vi "Itest.vi"() -> ()   [LabVIEW 2024]
uses:
  <vilib>/Analysis/baseanly.llb/Mean (DBL).vi
  <instrlib>/EFmeter/EFmeter.lvlib
  <vilib>/Analysis/NI_AALBase.lvlib
  BK Precision 8500B Series/BK Precision 8500B Series.lvlib
  Keithley DMM6500 DAQ6500 Series.lvlib
panel:
  in  "VISA DMM":refnum<visa-resource-name>
  in  "Zdroj":u16(ring) items=["Manualni", "K 2200"]
  out "error out 2":errorcluster
  in  "VISA EFmeter":refnum<visa-resource-name>
  out "R_out":dbl
  in  "file path (use dialog)":path
  in  "Prodleva mezi vzorky":u32
  out "napeti":dbl=2.5
  in  "velikost kroku":dbl
  in  "start":dbl
  in  "Prumerovani":bool
  in  "Vzorku na krokù":u16 max=100 step=1
  out "XY Graph 2":cluster{"X":dbl[], "Y":dbl[]}[](graph)
  in  "Pocet kroku":i32
  in  "Clear":bool
  in  "Uložit data":bool
  in  "Start":bool
  in  "VISA ZATEZ":refnum<visa-resource-name>
  in  "stop":bool
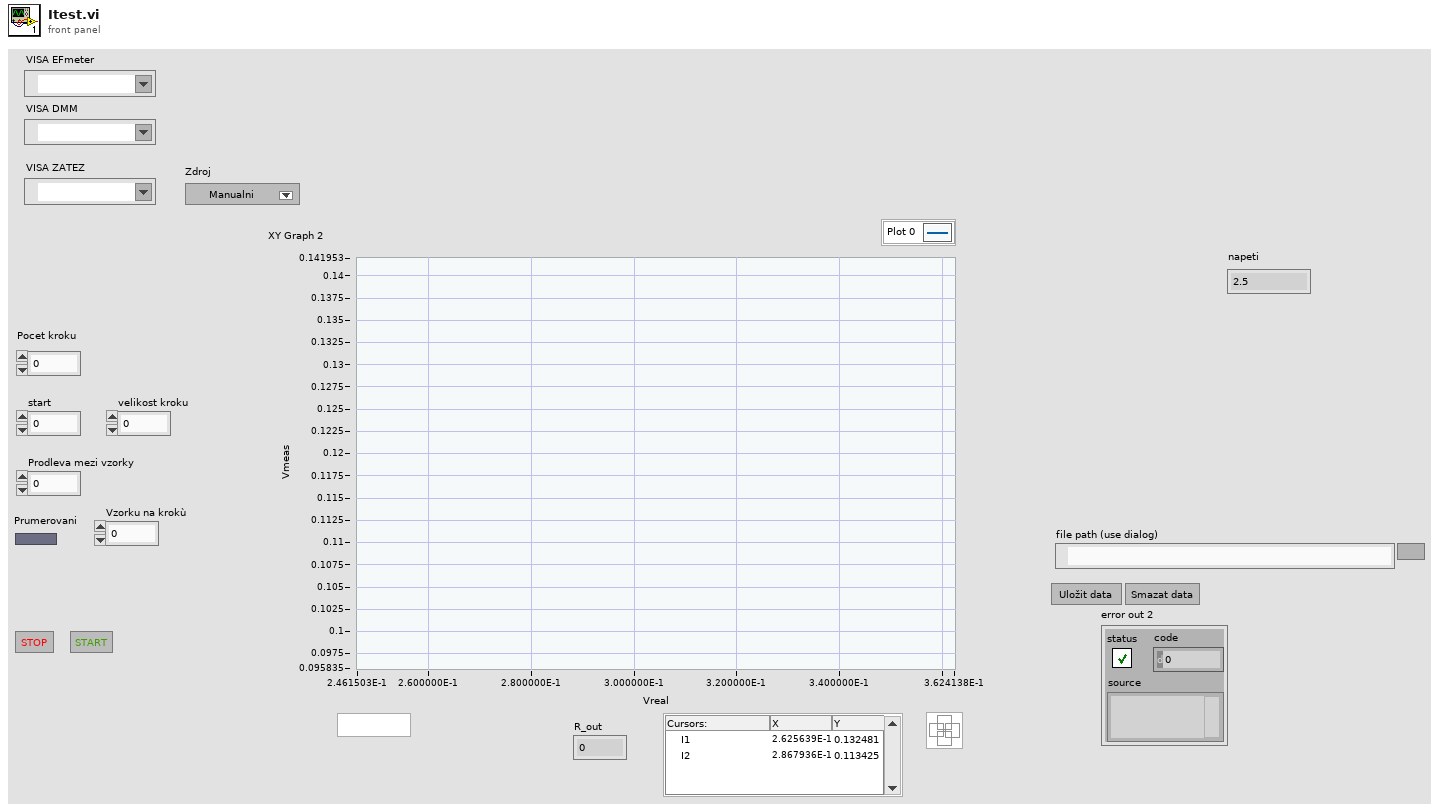
[diagram p1: front panel]
types:
  T1 = enum16{"init", "wait", "graph", "meas", "change_load", "init_measurment", "save", "clear"}
  T2 = typedef "LVCursorListTypeDef.ctl" = cluster{"Name":string, "Color":u32, "Style":u8, "Point Style":u8, "Name Visible":bool, "Allow Drag":bool, "Cursor Mode":u32, "Plot":i32, "Index":i32, "Position":cluster{"X":dbl, "Y":dbl}, "X Scale":u32, "Y Scale":u32, "Watch Plots":i32[], "Watch All Plots":bool, "Plot Area":i32, "Label Offset":cluster{"X":dbl, "Y":dbl}}[]
  T3 = cluster{"Name":string, "Color":u32, "Style":u8, "Point Style":u8, "Name Visible":bool, "Allow Drag":bool, "Cursor Mode":u32, "Plot":i32, "Index":i32, "Position":cluster{"X":dbl, "Y":dbl}, "X Scale":u32, "Y Scale":u32, "Watch Plots":i32[], "Watch All Plots":bool, "Plot Area":i32, "Label Offset":cluster{"X":dbl, "Y":dbl}}
  T4 = enum16{"open", "replace", "create", "open or create", "replace or create", "replace or create with confirmation"}
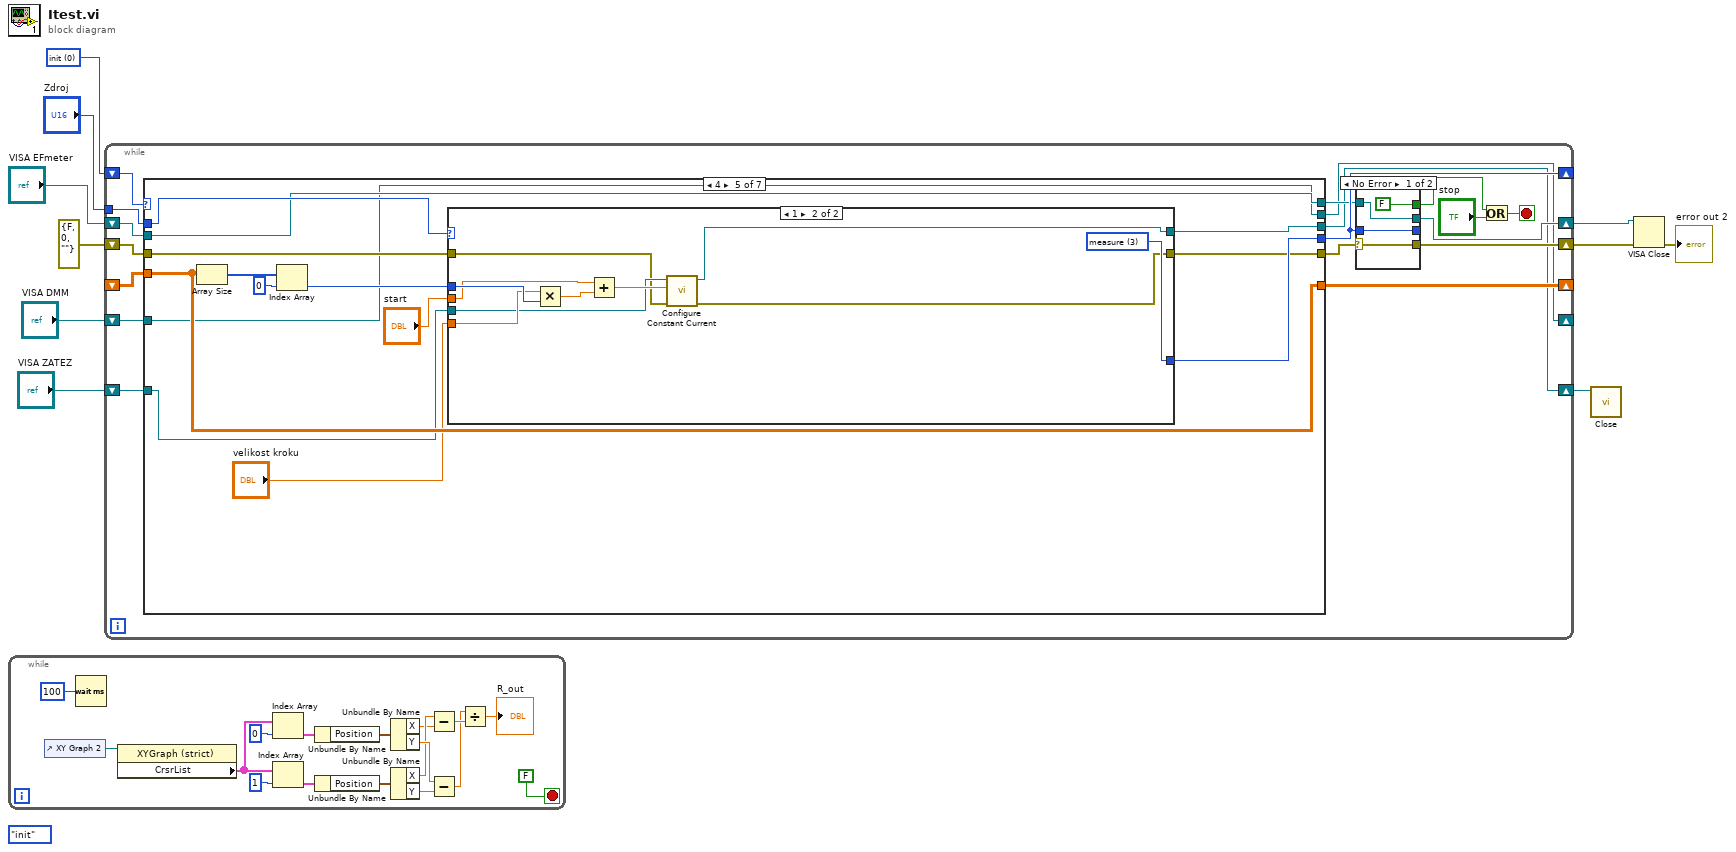
[diagram p0: block diagram]
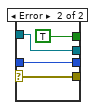
[diagram p2: hidden frame]
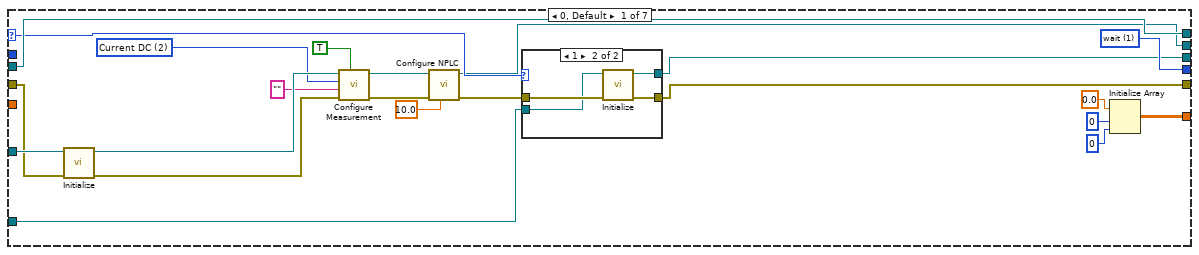
[diagram p3: hidden frame]
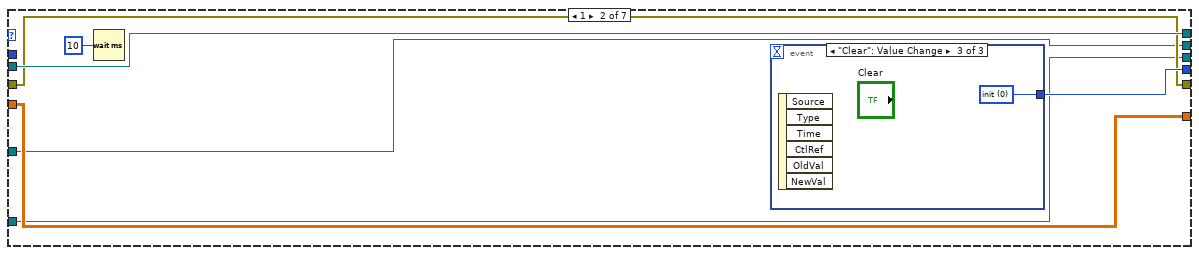
[diagram p5: hidden frame]
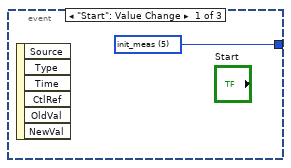
[diagram p6: hidden frame]
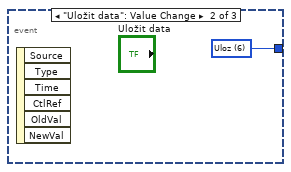
[diagram p7: hidden frame]
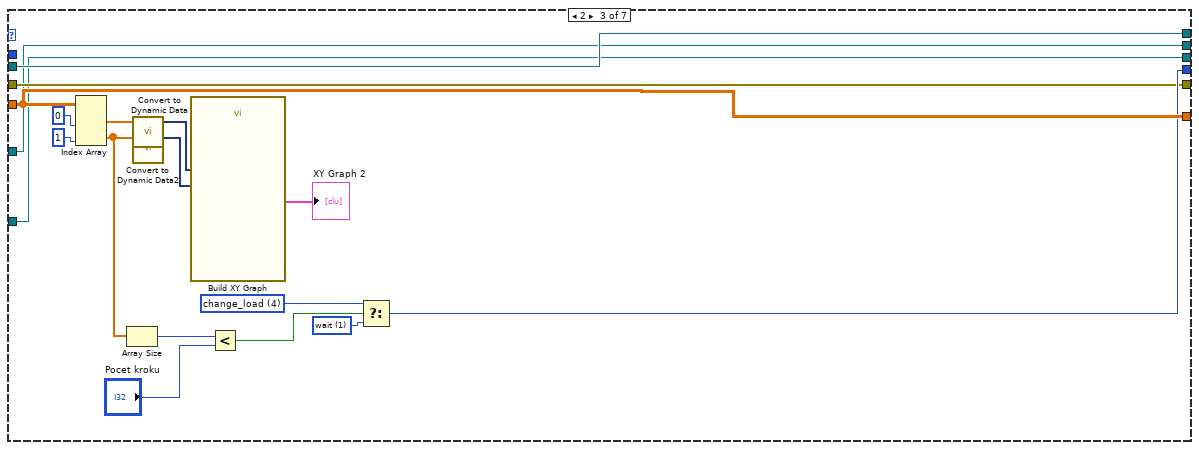
[diagram p8: hidden frame]
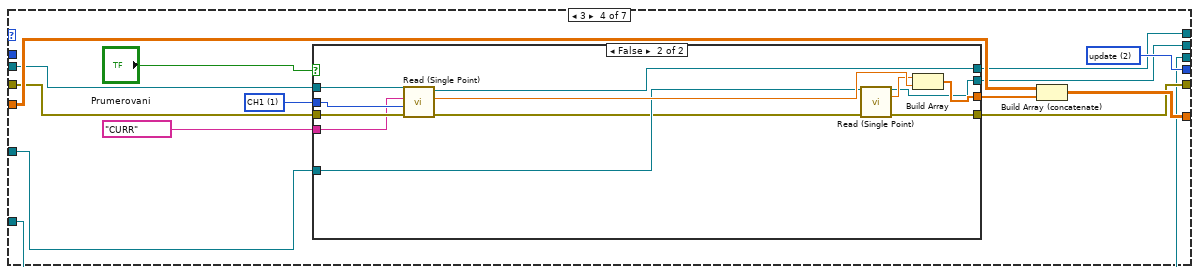
[diagram p9: hidden frame]
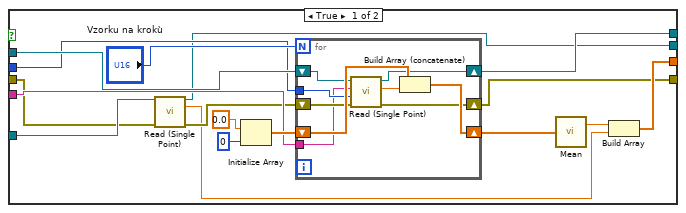
[diagram p10: hidden frame]
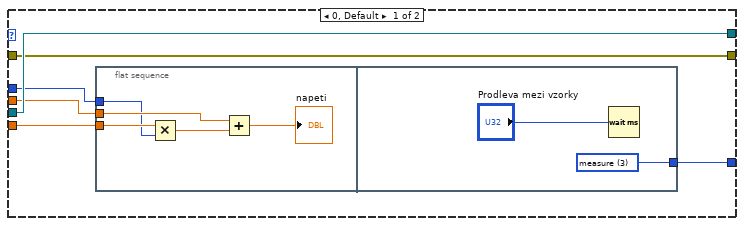
[diagram p11: hidden frame]
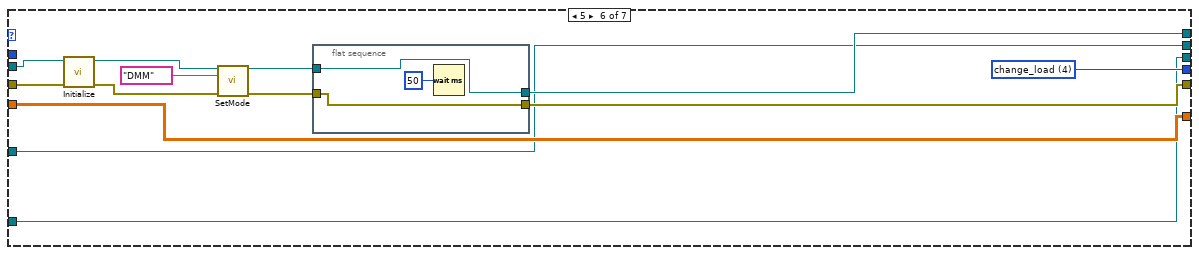
[diagram p12: hidden frame]
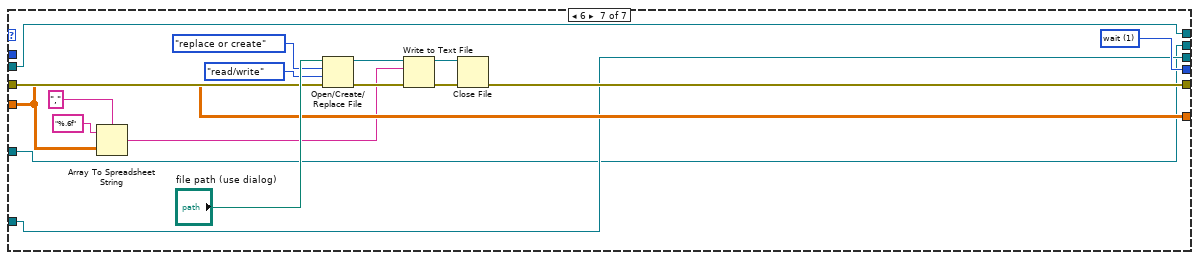
[diagram p13: hidden frame]
diagram:
  (unwired) T1."init"
  w10 = u16 0 items=["init", "wait", "update", "measure", "change_load", "init_meas", "Uloz", "clear"]
  n1 = while {
    stop <- FALSE stop-if-true
    n2 = control-ref of="XY Graph 2"() -> (w25:refnum<vi>)
    n3 = Wait (ms)(milliseconds to wait=u32 100) -> ()  [unwired: 1 out]
    n4 = property class="XYGraph (strict)"(reference=w25) -> ("CrsrList"=w20:T2)  [unwired: 1 in, 2 out]
    n5 = Index Array(array=w20, index=0) -> (element=w26:T3)
    n6 = Index Array(array=w20, index=1) -> (element=w22:T3)
    n7 = Unbundle By Name(w26) -> ("Position"=w27:cluster{"X":dbl, "Y":dbl})
    n8 = Unbundle By Name(w22) -> ("Position"=w23:cluster{"X":dbl, "Y":dbl})
    n9 = Unbundle By Name(w27) -> ("X"=w11:dbl, "Y"=w18:dbl)
    n10 = Unbundle By Name(w23) -> ("X"=w12:dbl, "Y"=w19:dbl)
    n11 = Subtract(x=w12, y=w11) -> (x-y=w14:dbl)
    n12 = Subtract(x=w18, y=w19) -> (x-y=w13:dbl)
    n13 = Divide(x=w13, y=w14) -> (x/y=→"R_out":dbl)
  }
  n14 = while {
    shift-right: [w45] -> _
    shift-left: _ -> [w44]
    shift-right: [w40] -> _
    shift-left: w10 -> [w43]
    shift-right: [w37] -> w6
    shift-left: "VISA EFmeter" -> [w42]
    shift-right: [w36] -> w5
    shift-left: errorcluster {"status"=FALSE, "code"=0, "source"=""} ("error in (no error)") -> [w41]
    tunnel: "Zdroj" -> [w32]
    shift-right: [w31] -> w3
    shift-left: "VISA ZATEZ" -> [w30]
    shift-right: [w28] -> _
    shift-left: "VISA DMM" -> [w29]
    stop <- w34 stop-if-true
    n15 = case shown="4" w43 {
      selector: w43 -> [w69 _ _ _ _ _ _]
      tunnel: [w73 w87 w101 w122 w175 w211 w226] -> w45
      tunnel: w44 -> [_ w87 w101 w123 w175 w211 w226]
      tunnel: [w72 w88 w100 w120 w173 w205 w224] -> w40
      tunnel: [w68 w85 w94 w114 w163 w202 w220] -> w39
      tunnel: [w70 w86 w95 w115 w172 w204 w231] -> w38
      tunnel: w42 -> [w70 w86 w95 w119 w172 w207 w231]
      tunnel: w41 -> [w64 w85 w94 w118 w164 w206 w227]
      tunnel: w32 -> [_ _ _ _ w174 _ _]
      tunnel: [w67 w83 w93 w112 w170 w200 w216] -> w31
      tunnel: w30 -> [w66 w83 w93 w112 w171 w200 w216]
      tunnel: w29 -> [w65 w82 w92 w111 w162 w199 w215]
      tunnel: [w55 w82 w92 w110 w162 w199 w215] -> w28
      frame 0, Default {
        w61 = 2 items=["Voltage DC", "Voltage AC", "Current DC", "Current AC", "Resistance", "4-wire Resistance", "Diode", "Capacitance", "Temperature", "Continuity", "Frequency", "Period", "Voltage Ratio", "Digitize Voltage", "Digitize Current"] ("Function (0: Voltage DC)")
        w72 = u16 1 items=["init", "wait", "update", "measure"]
        n16 = call "Initialize.vi"("error in (no error)"=w64, "VISA resource name"=w65) -> ("error out"=w63:errorcluster, "VISA resource name out"=w62:refnum<visa-resource-name>)  [unwired: 8 in]
        n17 = call "Configure Measurement.vi"("Auto Range (T: Enable)"=TRUE, "error in (no error)"=w63, "Channel List(\"\")"="" ("Channel List(\"\")"), "Function (0: Voltage DC)"=w61, "VISA resource name"=w62) -> ("error out"=w56:errorcluster, "VISA resource name out"=w57:refnum<visa-resource-name>)  [unwired: 5 in]
        n18 = call "Configure NPLC.vi"("Power Line Cycle (1)"=10.0, "error in (no error)"=w56, "VISA resource name"=w57) -> ("error out"=w54:errorcluster, "VISA resource name out"=w55:refnum<visa-resource-name>)  [unwired: 7 in]
        n19 = case shown="1" w69 {
          tunnel: w54 -> [w77 w81]
          tunnel: [w77 w78] -> w68
          tunnel: [w76 w79] -> w67
          tunnel: w66 -> [w76 w80]
          frame 0, Default {
          }
          frame 1 {
            n20 = call "Initialize.vi"("error in (no error)"=w81, "VISA resource name"=w80) -> ("error out"=w78:errorcluster, "VISA resource name out"=w79:refnum<visa-resource-name>)  [unwired: 8 in]
          }
        }
        n21 = Initialize Array(0.0 ("element"), 0 ("dimension size"), 0 ("dimension size")) -> (w73:dbl[][])
      }
      frame 1 {
        n22 = Wait (ms)(milliseconds to wait=u32 10) -> ()  [unwired: 1 out]
        n23 = event shown="[2] \"Clear\": Value Change" {
          selector: _ -> [_ _ _]
          dyn-events: _ -> [_ _ _]
          timeout: _ -> [_ _ _]
          tunnel: [w89 w90 w91] -> w88
          event "Start": Value Change {
            w89 = u16 5 items=["init", "wait", "update", "measure", "change_load", "init_meas"]
            n24 = event-data() -> ()  [unwired: 1 in, 6 out]
          }
          event "Uložit data": Value Change {
            w90 = u16 6 items=["init", "wait", "update", "measure", "change_load", "init_meas", "Uloz"]
            n25 = event-data() -> ()  [unwired: 1 in, 6 out]
          }
          event "Clear": Value Change {
            w91 = u16 0 items=["init", "wait", "update", "measure", "change_load", "init_meas", "Uloz", "clear"]
            n26 = event-data() -> ()  [unwired: 1 in, 6 out]
          }
        }
      }
      frame 2 {
        w96 = u16 4 items=["init", "wait", "update", "measure", "change_load", "init_meas"]
        w102 = u16 1 items=["init", "wait", "update", "measure"]
        n27 = Index Array(array=w101, index (col) #1=0 ("index (row)"), index (col) #2=1 ("index (row)")) -> (element #1=w109:dbl[], element #2=w104:dbl[])  [unwired: 2 in]
        n28 = Array Size(array=w104) -> (size(s)=w106:i32)
        n29 = call "Convert to Dynamic Data"("Array"=w109) -> ("Dynamic Data Type"=w108:dynamicdata)  [unwired: 3 in]
        n30 = call "Convert to Dynamic Data2"("Array"=w104) -> ("Dynamic Data Type"=w107:dynamicdata)  [unwired: 3 in]
        n31 = call "Build XY Graph"("Y Input"=w107, "X Input"=w108) -> ("XY Graph"=→"XY Graph 2":cluster{"X":dbl[], "Y":dbl[]}[])  [unwired: 8 in, 1 out]
        n32 = Less?(x=w106, y="Pocet kroku") -> (x < y?=w105:bool)
        n33 = Select(t=w96, s=w105, f=w102) -> (s? t:f=w100:u16)
      }
      frame 3 {
        w117 = u16 1 items=["CH2"=2, "CH1"=1] ("Ring")
        w120 = u16 2 items=["init", "wait", "update", "measure"]
        n34 = case shown="False" "Prumerovani" {
          tunnel: [w132 w161] -> w121
          tunnel: w119 -> [w136 w160]
          tunnel: w118 -> [w127 w159]
          tunnel: w117 -> [w135 w158]
          tunnel: "CURR" ("Combo Box") -> [w134 w157]
          tunnel: [w131 w152] -> w115
          tunnel: [w130 w153] -> w114
          tunnel: w111 -> [w129 w155]
          tunnel: [w128 w150] -> w110
          frame True {
            n35 = call "Read (Single Point).vi"("VISA resource name"=w129, "error in (no error)"=w127) -> ("VISA resource name out"=w128:refnum<visa-resource-name>, "Measurement"=w125:dbl, "error out"=w126:errorcluster)  [unwired: 11 in]
            n36 = Initialize Array(0.0 ("element"), 0 ("dimension size")) -> (w137:dbl[])
            n37 = for {
              N: "Vzorku na krokù" -> [_]
              shift-right: [w142] -> w131
              shift-left: w136 -> [w148]
              shift-right: [w143] -> w130
              shift-left: w126 -> [w147]
              tunnel: w135 -> [w146]
              tunnel: w134 -> [w145]
              shift-right: [w144] -> w124
              shift-left: w137 -> [w149]
              n38 = call "Read (Single Point).vi"("error in (no error)"=w147, "Ring"=w146, "Combo Box"=w145, "VISA resource name"=w148) -> ("error out"=w143:errorcluster, "Measurement"=w141:dbl, "VISA resource name out"=w142:refnum<visa-resource-name>)  [unwired: 5 in]
              n39 = Build Array (concatenate)(w149, w141) -> (w144:dbl[])
            }
            n40 = call-poly <vilib>:"Mean.vi"("X"=w124) -> ("mean"=w133:dbl)  [unwired: 1 out]
            n41 = Build Array(w133, w125) -> (w132:dbl[])
          }
          frame False {
            n42 = call "Read (Single Point).vi"("error in (no error)"=w159, "Ring"=w158, "Combo Box"=w157, "VISA resource name"=w160) -> ("error out"=w154:errorcluster, "Measurement"=w156:dbl, "VISA resource name out"=w152:refnum<visa-resource-name>)  [unwired: 5 in]
            n43 = call "Read (Single Point).vi"("VISA resource name"=w155, "error in (no error)"=w154) -> ("VISA resource name out"=w150:refnum<visa-resource-name>, "Measurement"=w151:dbl, "error out"=w153:errorcluster)  [unwired: 11 in]
            n44 = Build Array(w151, w156) -> (w161:dbl[])
          }
        }
        n45 = Build Array (concatenate)(w123, w121) -> (w122:dbl[][])
      }
      frame 4 {
        n46 = Array Size(array=w175) -> (size(s)=w165:i32[])
        n47 = Index Array(array=w165, index=0) -> (element=w167:i32)
        n48 = case shown="1" w174 {
          tunnel: [w181 w198] -> w173
          tunnel: w171 -> [w180 w190]
          tunnel: [w180 w193] -> w170
          tunnel: "velikost kroku" -> [w179 w196]
          tunnel: "start" -> [w178 w194]
          tunnel: w167 -> [w177 w197]
          tunnel: w164 -> [w176 w189]
          tunnel: [w176 w192] -> w163
          frame 0, Default {
            n49 = flat-sequence {
              tunnel: w179 -> [w184]
              tunnel: w178 -> [w183]
              tunnel: w177 -> [w182]
              tunnel: [w187] -> w181
              frame #0 {
                n50 = Multiply(x=w184, y=w182) -> (x*y=w186:dbl)
                n51 = Add(x=w183, y=w186) -> (x+y=→"napeti":dbl)
              }
              frame #1 {
                w187 = u16 3 items=["init", "wait", "update", "measure", "change_load", "init_meas"]
                n52 = Wait (ms)(milliseconds to wait="Prodleva mezi vzorky") -> ()  [unwired: 1 out]
              }
            }
          }
          frame 1 {
            w198 = u16 3 items=["init", "wait", "update", "measure", "change_load", "init_meas"]
            n53 = Multiply(x=w196, y=w197) -> (x*y=w195:dbl)
            n54 = Add(x=w194, y=w195) -> (x+y=w191:dbl)
            n55 = call "Configure Constant Current.vi"("error in (no error)"=w189, "CC Current (0)"=w191, "VISA resource name"=w190) -> ("error out"=w192:errorcluster, "VISA resource name out"=w193:refnum<visa-resource-name>)  [unwired: 7 in]
          }
        }
      }
      frame 5 {
        w205 = u16 4 items=["init", "wait", "update", "measure", "change_load", "init_meas"]
        n56 = call "Initialize.vi"("error in (no error)"=w206, "VISA resource name"=w207) -> ("error out"=w210:errorcluster, "VISA resource name out"=w209:refnum<visa-resource-name>)  [unwired: 8 in]
        n57 = call "SetMode.vi"("VISA resource name"=w209, "Combo Box"="DMM", "error in (no error)"=w210) -> ("VISA resource name out"=w203:refnum<visa-resource-name>, "error out"=w201:errorcluster)  [unwired: 11 in]
        n58 = flat-sequence {
          tunnel: [w213] -> w204
          tunnel: w203 -> [w213]
          tunnel: w201 -> [w212]
          tunnel: [w212] -> w202
          frame #0 {
            n59 = Wait (ms)(milliseconds to wait=u32 50) -> ()  [unwired: 1 out]
          }
        }
      }
      frame 6 {
        w224 = u16 1 items=["init", "wait", "update", "measure", "change_load", "init_meas"]
        n60 = Array To Spreadsheet String(delimiter (Tab)=",", array=w226, 3:"%.6f" ("format string")) -> (spreadsheet string=w217:string)
        n61 = Open/Create/Replace File(file path (use dialog)="file path (use dialog)", error in=w227, operation (0:open)=T4."replace or create", access (0:read/write)=enum16{"read/write", "read-only", "write-only"}."read/write") -> (refnum out=w219:refnum<file>, error out=w222:errorcluster)  [unwired: 2 in, 1 out]
        n62 = Write to Text File(file (use dialog)=w219, text=w217, error in=w222) -> (refnum out=w218:refnum<file>, error out=w221:errorcluster)  [unwired: 1 in, 1 out]
        n63 = Close File(refnum=w218, error in=w221) -> (error out=w220:errorcluster)  [unwired: 1 out]
      }
    }
    n64 = case shown="No Error" w39 {
      selector: w39 -> [w47 w51]
      tunnel: w40 -> [w49 w52]
      tunnel: [w49 w52] -> _
      tunnel: w38 -> [w48 w53]
      tunnel: [w48 w53] -> w37
      tunnel: [w47 w51] -> w36
      tunnel: [FALSE TRUE] -> w33
      frame No Error {
      }
      frame Error {
      }
    }
    n65 = Or(x=w33, y="stop") -> (x .or. y?=w34:bool)
  }
  n66 = call "Close.vi"("VISA resource name"=w3) -> ()  [unwired: 10 in, 1 out]
  n67 = VISA Close(VISA resource name=w6, error in (no error)=w5) -> (error out=→"error out 2":errorcluster)
